vi "SmartSEM Remote API get string.vi"(8 "error in":errorcluster, 10 "lpszParam":string, 11 "Api":refnum<k7>(container)) -> (0 "error out":errorcluster, 2 "data":string, 3 "Api out":refnum<k7>)   [LabVIEW 2018]
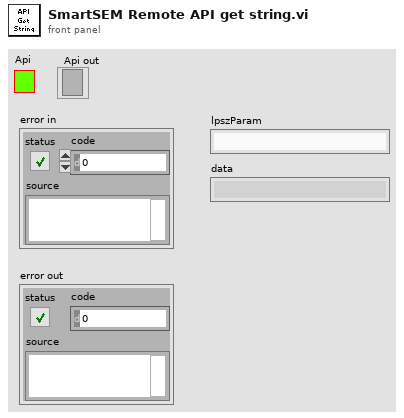
[diagram p1: front panel]
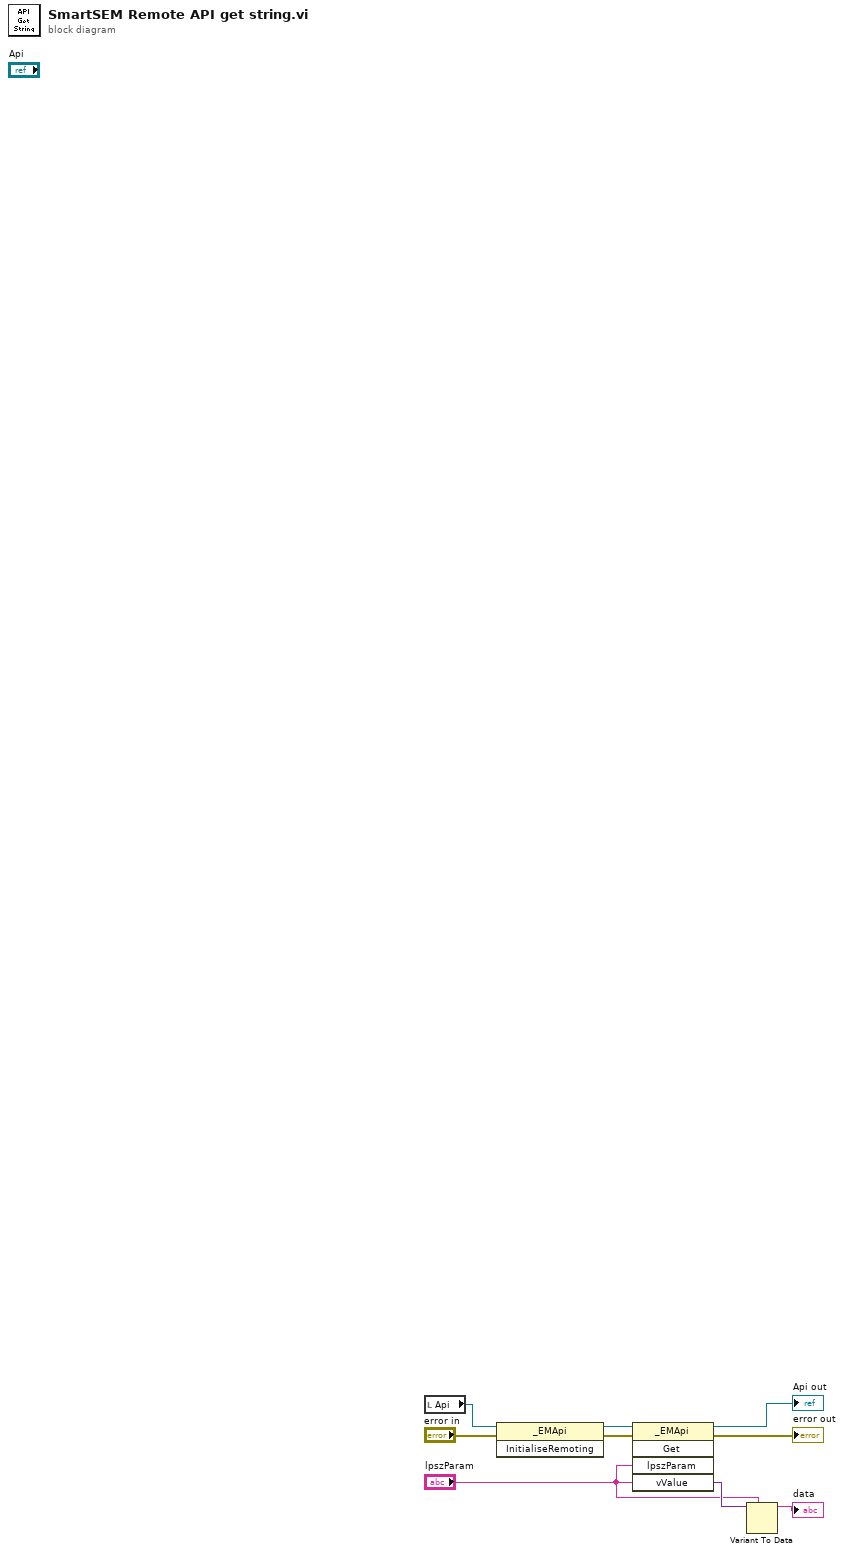
[diagram p0: block diagram]
diagram:
  n1 = local read "Api"() -> (w9:refnum<k7>)
  n2 = invoke class="_EMApi" method="InitialiseRemoting"(reference=w9, error in="error in") -> (reference out=w4:refnum<k7>, error out=w3:errorcluster)  [unwired: 1 in, 1 out]
  n3 = invoke class="_EMApi" method="Get"(reference=w4, error in=w3, "lpszParam"="lpszParam", "vValue"="lpszParam") -> (reference out=→"Api out":refnum<k7>, error out=→"error out":errorcluster, "vValue"=w5:variant)  [unwired: 1 in, 2 out]
  n4 = Variant To Data(type="lpszParam", Variant=w5) -> (data=→"data":string)  [unwired: 1 in, 1 out]
